vi "Lab view.vi"() -> ()   [LabVIEW 2020]
panel:
  out "Fire indicator":bool
  in  "VISA resource name":refnum<visa-resource-name>
  out "Smoke":bool
  out "Flame":bool
  in  "Table Control":string[][](table)
  out "Smoke Chart":i32(graph)
  out "Flame Chart":i32(graph)
  out "SMOKE":dbl(slide) scale=0.0..100.0
  out "FLAME":dbl(slide) scale=0.0..100.0
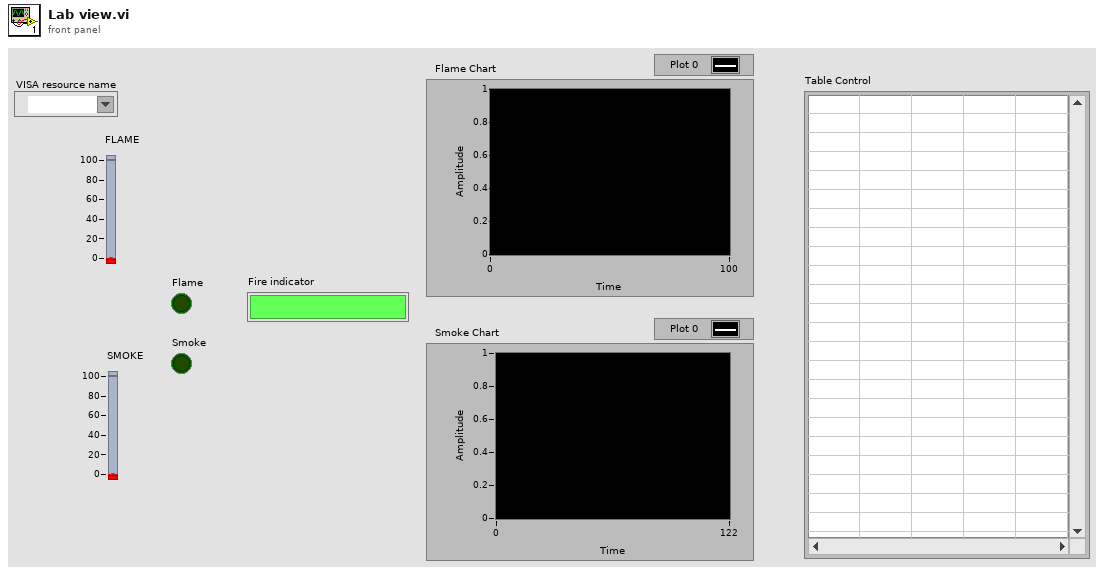
[diagram p1: front panel]
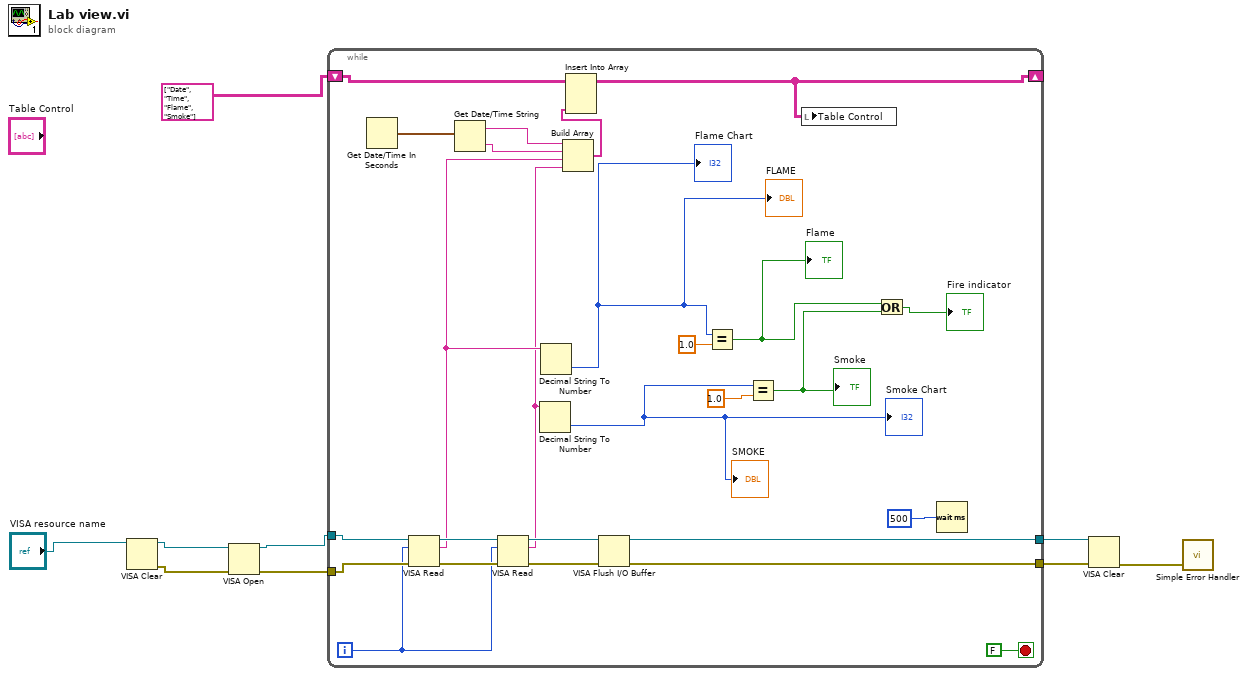
[diagram p0: block diagram]
diagram:
  n1 = VISA Clear(VISA resource name="VISA resource name") -> (VISA resource name out=w8:refnum<visa-resource-name>, error out=w7:errorcluster)  [unwired: 1 in]
  n2 = VISA Open(error in (no error)=w7, VISA resource name=w8) -> (VISA resource name=w6:refnum<visa-resource-name>, error out=w5:errorcluster)  [unwired: 3 in]
  n3 = while {
    tunnel: w6 -> [w33]
    tunnel: w5 -> [w32]
    tunnel: [w29] -> w4
    tunnel: [w28] -> w3
    shift-right: [w10] -> _
    shift-left: string[][] [["Date", "Time", "Flame", "Smoke"]] ("Table Control") -> [w11]
    i -> [w12]
    stop <- FALSE stop-if-true
    n4 = Get Date/Time In Seconds() -> (seconds since 1Jan1904=w27:timestamp)
    n5 = VISA Read(VISA resource name=w33, byte count=w12, error in (no error)=w32) -> (VISA resource name out=w31:refnum<visa-resource-name>, read buffer=w22:string, error out=w24:errorcluster)  [unwired: 1 out]
    n6 = Get Date/Time String(seconds (now)=w27) -> (date string=w25:string, time string=w26:string)  [unwired: 2 in]
    n7 = VISA Read(VISA resource name=w31, byte count=w12, error in (no error)=w24) -> (VISA resource name out=w30:refnum<visa-resource-name>, read buffer=w21:string, error out=w23:errorcluster)  [unwired: 1 out]
    n8 = Decimal String To Number(string=w21) -> (number=w17:i32)  [unwired: 2 in, 1 out]
    "SMOKE" <- w17
    "Smoke Chart" <- w17
    n9 = Decimal String To Number(string=w22) -> (number=w16:i32)  [unwired: 2 in, 1 out]
    "Flame Chart" <- w16
    "FLAME" <- w16
    n10 = Build Array(w25, w26, w22, w21) -> (w20:string[])
    n11 = Insert Into Array(array=w11, new element=w20) -> (w10:string[][])  [unwired: 2 in]
    n12 = VISA Flush I/O Buffer(VISA resource name=w30, error in (no error)=w23) -> (VISA resource name out=w29:refnum<visa-resource-name>, error out=w28:errorcluster)  [unwired: 1 in]
    n13 = Equal?(x=w16, y=1.0) -> (x = y?=w14:bool)
    "Flame" <- w14
    n14 = Equal?(x=w17, y=1.0) -> (x = y?=w15:bool)
    "Smoke" <- w15
    n15 = local write "Table Control"(w10) -> ()
    n16 = Or(x=w14, y=w15) -> (x .or. y?=→"Fire indicator":bool)
    n17 = Wait (ms)(milliseconds to wait=u32 500) -> ()  [unwired: 1 out]
  }
  n18 = VISA Clear(VISA resource name=w4, error in (no error)=w3) -> (error out=w2:errorcluster)  [unwired: 1 out]
  n19 = call <vilib>:"Simple Error Handler.vi"("error in (no error)"=w2) -> ()  [unwired: 4 in, 5 out]
